vi "PushVal2Disabled.vi"(6 "Value":string, 8 "error in (no error)":errorcluster, 10 "Cell Position":T1, 11 "Table CtlRef In":refnum<vi>) -> (0 "error out":errorcluster, 2 "pushed?":bool, 3 "Table CtlRef Out":refnum<vi>)   [LabVIEW 2013]
uses:
  <vilib>/Utility/miscctls.llb/LVRowAndColumnTypeDef.ctl
  Globals/DisabledColorGlobal.vi
panel:
  out "# pushed":i32
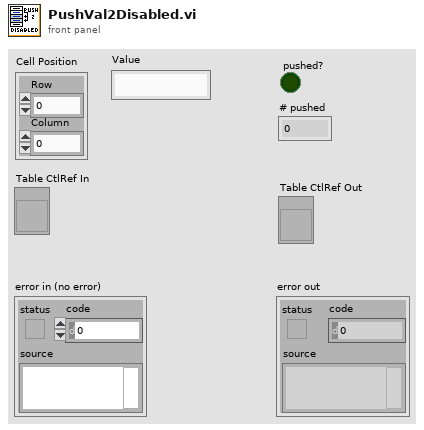
[diagram p1: front panel]
types:
  T1 = typedef "LVRowAndColumnTypeDef.ctl" = cluster{"Row":i32, "Column":i32}
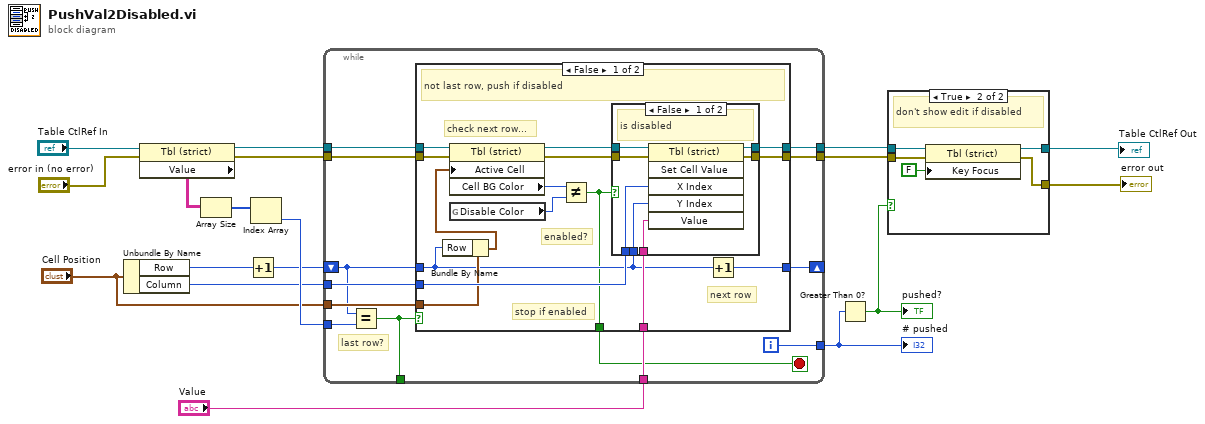
[diagram p0: block diagram]
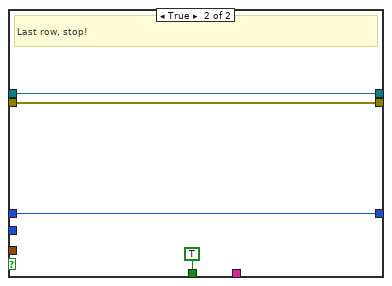
[diagram p4: hidden frame]
diagram:
  n1 = Unbundle By Name("Cell Position") -> ("Row"=w13:i32, "Column"=w11:i32)
  n2 = property class="Tbl (strict)"(reference="Table CtlRef In", error in="error in (no error)") -> (reference out=w10:refnum<vi>, error out=w9:errorcluster, "Value"=w16:string[][])
  n3 = Array Size(array=w16) -> (size(s)=w15:i32[])
  n4 = Increment(x=w13) -> (x+1=w12:i32)
  n5 = Index Array(array=w15) -> (element=w14:i32)  [unwired: 1 in]
  n6 = while {
    tunnel: w14 -> [w31]
    shift-right: [w30] -> _
    shift-left: w12 -> [w21]
    tunnel: w11 -> [w25]
    tunnel: w10 -> [w29]
    tunnel: w9 -> [w28]
    tunnel: [w27] -> w2
    tunnel: [w26] -> w1
    tunnel: "Value" -> [w24]
    tunnel: "Cell Position" -> [w23]
    tunnel: [w22] -> w6
    tunnel: [w19] -> _
    i -> [w22]
    stop <- w20 stop-if-true
    # "last row?"
    n7 = Equal?(x=w21, y=w31) -> (x = y?=w19:bool)
    n8 = case shown="False" w19 {
      tunnel: [w46 w57] -> w30
      tunnel: w29 -> [w45 w59]
      tunnel: w28 -> [w44 w58]
      tunnel: [w39 w59] -> w27
      tunnel: [w38 w58] -> w26
      tunnel: w25 -> [w37 _]
      tunnel: w24 -> [w36 _]
      tunnel: w23 -> [w35 _]
      tunnel: w21 -> [w33 w57]
      tunnel: [w32 TRUE] -> w20
      frame False {
        # "check next row..."
        # "stop if enabled"
        # "enabled?"
        # "next row"
        # "not last row, push if disabled"
        n9 = Bundle By Name(cluster=w35, "Row"=w33) -> (w34:T1)
        n10 = property class="Tbl (strict)"(reference=w45, error in=w44, "Active Cell"=w34) -> (reference out=w41:refnum<vi>, error out=w40:errorcluster, "Cell BG Color"=w43:u32)
        n11 = global read "DisabledColorGlobal.vi" "Disable Color"() -> (w42:u32)
        n12 = Not Equal?(x=w43, y=w42) -> (x != y?=w32:bool)
        n13 = case shown="False" w32 {
          tunnel: w41 -> [w53 w55]
          tunnel: w40 -> [w52 w54]
          tunnel: [w51 w55] -> w39
          tunnel: [w50 w54] -> w38
          tunnel: w33 -> [w49 _]
          tunnel: w37 -> [w48 _]
          tunnel: w36 -> [w47 _]
          frame False {
            # "is disabled"
            n14 = invoke class="Tbl (strict)" method="Set Cell Value"(reference=w53, error in=w52, "X Index"=w48, "Y Index"=w49, "Value"=w47) -> (reference out=w51:refnum<vi>, error out=w50:errorcluster)  [unwired: 1 in, 4 out]
          }
          frame True {
            # "not disabled"
          }
        }
        n15 = Increment(x=w33) -> (x+1=w46:i32)
      }
      frame True {
        # "Last row, stop!"
      }
    }
  }
  "# pushed" <- w6
  n16 = Greater Than 0?(x=w6) -> (x > 0?=w5:bool)
  "pushed?" <- w5
  n17 = case shown="True" w5 {
    tunnel: w2 -> [w61 w66]
    tunnel: [w61 w65] -> w3
    tunnel: w1 -> [w60 w64]
    tunnel: [w60 w63] -> w4
    frame False {
    }
    frame True {
      # "don't show edit if disabled"
      n18 = property class="Tbl (strict)"(reference=w66, error in=w64, "Key Focus"=FALSE) -> (reference out=w65:refnum<vi>, error out=w63:errorcluster)
    }
  }
  "error out" <- w4
  "Table CtlRef Out" <- w3
